vi "Config Math.vi"(0 "VISA resource name":refnum<visa-resource-name>, 1 "Math1 (F: OFF)":bool, 2 "Math1 Expression (C1)":string="C1", 3 "Math1 Unit (V)":string="V", 5 "Math Mode (F: OFF)":bool, 7 "Start Point (0)":dbl min=0.0 format="%.2f", 9 "End Point (0)":dbl min=0.0 format="%.2f", 11 "error in (no error)":errorcluster, 12 "Math2 (F: OFF)":bool, 13 "Math2 Expression (C2)":string="C2", 14 "Math2 Unit (A)":string="A") -> (4 "VISA resource name out":refnum<visa-resource-name>, 15 "error out":errorcluster)   [LabVIEW 2013, in "Yokogawa.lvlib" / "Yokogawa PZ4000.lvlib"]
doc: "This VI sends the Math command to the PZ4000 series.\nConfigure Control Functions are Selects the Math Mode, Expression , Unit, Strat points and End points."
uses:
  Yokogawa PZ4000.lvlib
panel:
  # "ON\nOFF"
  # "ON\nOFF"
  # "ON\nOFF"
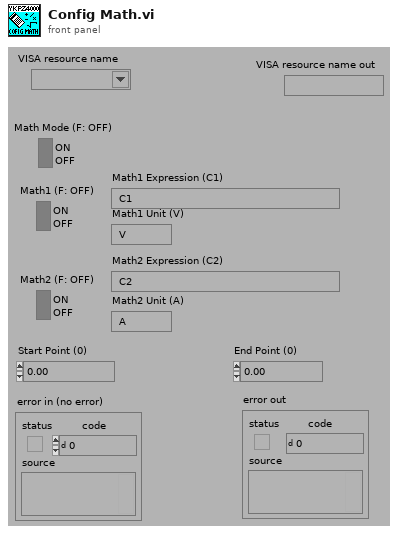
[diagram p1: front panel]
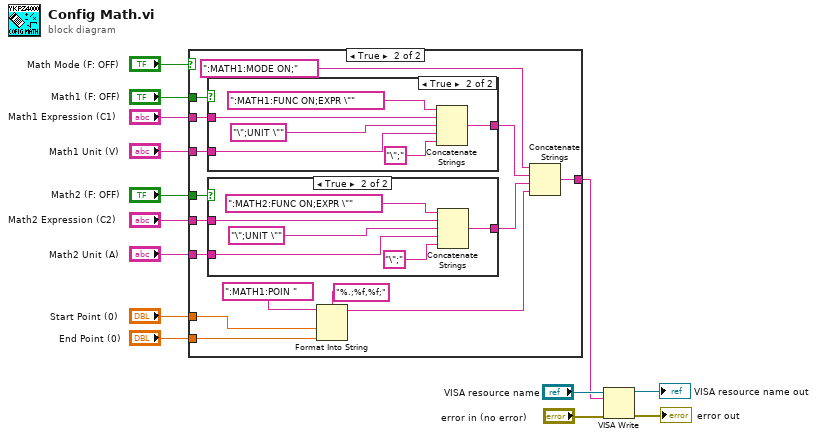
[diagram p0: block diagram]
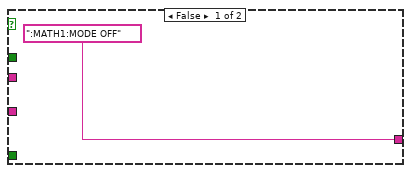
[diagram p2: hidden frame]
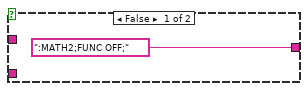
[diagram p3: hidden frame]
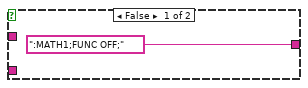
[diagram p4: hidden frame]
diagram:
  n1 = case shown="True" "Math Mode (F: OFF)" {
    tunnel: [":MATH1:MODE OFF" w17] -> w1
    tunnel: "Math1 (F: OFF)" -> [_ w30]
    tunnel: "Math2 (F: OFF)" -> [_ w27]
    tunnel: "Math1 Expression (C1)" -> [_ w29]
    tunnel: "Math1 Unit (V)" -> [_ w28]
    tunnel: "Math2 Expression (C2)" -> [_ w26]
    tunnel: "Math2 Unit (A)" -> [_ w25]
    tunnel: "Start Point (0)" -> [_ w19]
    tunnel: "End Point (0)" -> [_ w18]
    frame False {
    }
    frame True {
      n2 = case shown="True" w30 {
        tunnel: w29 -> [_ w43]
        tunnel: w28 -> [_ w41]
        tunnel: [":MATH1;FUNC OFF;" w40] -> w23
        frame False {
        }
        frame True {
          n3 = Concatenate Strings(":MATH1:FUNC ON;EXPR \"", w43, "\";UNIT \"", w41, "\";") -> (w40:string)
        }
      }
      n4 = case shown="True" w27 {
        tunnel: w26 -> [_ w35]
        tunnel: w25 -> [_ w34]
        tunnel: [":MATH2;FUNC OFF;" w33] -> w22
        frame False {
        }
        frame True {
          n5 = Concatenate Strings(":MATH2:FUNC ON;EXPR \"", w35, "\";UNIT \"", w34, "\";") -> (w33:string)
        }
      }
      n6 = Format Into String(format string="%.;%f,%f;", initial string=":MATH1:POIN ", w19, w18) -> (resulting string=w16:string)  [unwired: 1 in, 1 out]
      n7 = Concatenate Strings(":MATH1:MODE ON;", w23, w22, w16) -> (w17:string)
    }
  }
  n8 = VISA Write(VISA resource name="VISA resource name", write buffer=w1, error in (no error)="error in (no error)") -> (VISA resource name out=→"VISA resource name out":refnum<visa-resource-name>, error out=→"error out":errorcluster)  [unwired: 1 out]
